vi "Lim_Sup.vi"(8 "error in (no error)":errorcluster, 10 "Lim_Sup":u8, 11 "Contador_Bin_Actor in":refnum<class "Contador_Bin_Actor.lvclass">) -> (0 "error out":errorcluster, 3 "Contador_Bin_Actor out":refnum<class "Contador_Bin_Actor.lvclass">)   [LabVIEW 2019, in "Contador_Bin_Actor.lvlib" / "Contador_Bin_Actor.lvclass"]
uses:
  Contador_Bin_Actor.lvclass
  Contador_Bin_Actor.lvclass/Contador_Bin_Actor.ctl
  Aumentar_contador/Aumentar_contador Messages/Lim_Sup Msg/Lim_Sup Msg.lvclass/Lim_Sup Msg.ctl
  <vilib>/ActorFramework/Message Enqueuer/Message Enqueuer.lvclass/Message Enqueuer.ctl
  <vilib>/ActorFramework/Message Enqueuer/Enqueue.vi
  Aumentar_contador/Aumentar_contador Messages/Lim_Sup Msg/Lim_Sup Msg.lvclass
  C:/Program Files/National Instruments/LabVIEW 2019/vi.lib/ActorFramework/Message/Message.lvclass
  <vilib>/ActorFramework/Message Priority Queue/Priority Enqueue.vi
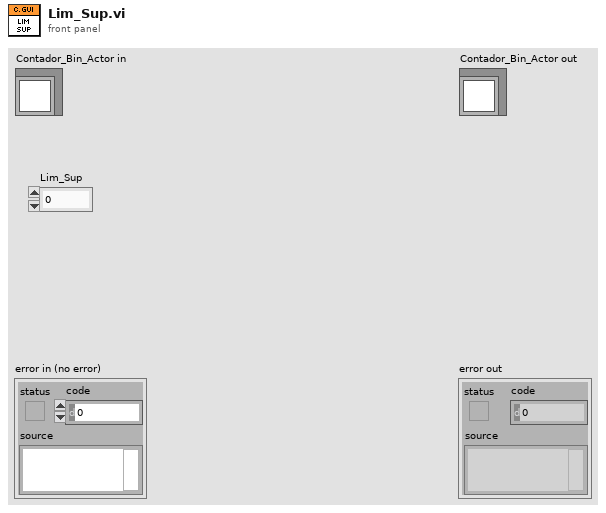
[diagram p1: front panel]
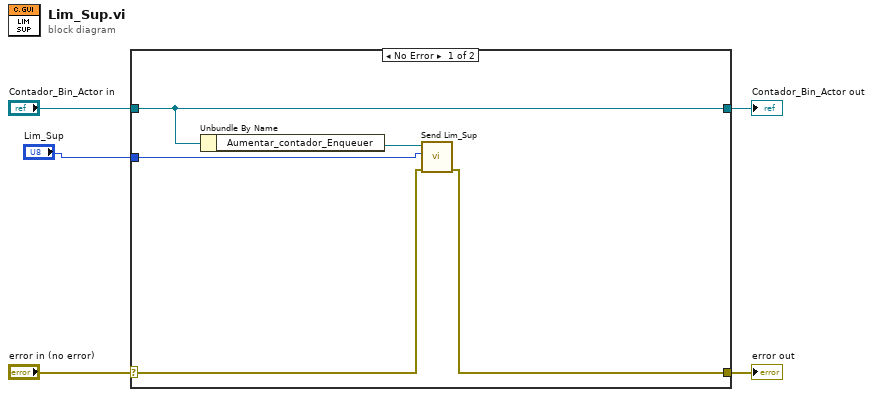
[diagram p0: block diagram]
diagram:
  n1 = case shown="No Error" "error in (no error)" {
    selector: "error in (no error)" -> [w8 w12]
    tunnel: [w7 w12] -> w4
    tunnel: [w10 w11] -> w2
    tunnel: "Contador_Bin_Actor in" -> [w10 w11]
    tunnel: "Lim_Sup" -> [w6 _]
    frame No Error {
      n2 = Unbundle By Name(w10) -> ("Aumentar_contador_Enqueuer"=w9:refnum<class "Message Enqueuer.lvclass">)
      n3 = call "Send Lim_Sup.vi"("error in (no error)"=w8, "Lim. Sup"=w6, "Message Enqueuer"=w9) -> ("error out"=w7:errorcluster)  [unwired: 7 in, 1 out]
    }
    frame Error {
    }
  }
  "error out" <- w4
  "Contador_Bin_Actor out" <- w2
